vi "Tosca-MATLAB Thread.vi"   [LabVIEW 2020]
uses:
  Typedefs/Tosca-MATLAB Queue Data.ctl
types:
  T1 = typedef "Tosca-MATLAB Queue Data.ctl" = cluster{"MATLAB function":path, "Datafile":path}
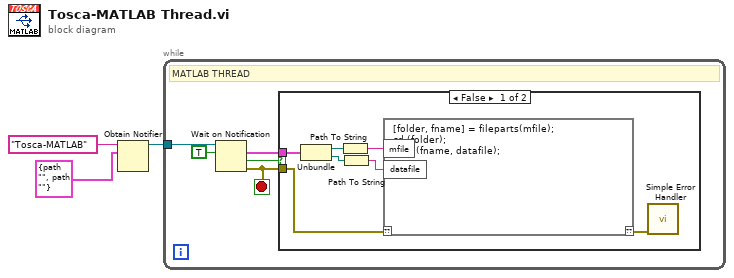
[diagram p0: block diagram]
diagram:
  n1 = Obtain Notifier(name (unnamed)="Tosca-MATLAB" ("Start"), notification data type=T1 {"MATLAB function"=path "", "Datafile"=path ""} ("Data")) -> (notifier out=w1:refnum<notifier>)  [unwired: 2 in, 2 out]
  n2 = while {
    tunnel: w1 -> [w8]
    stop <- w5 stop-if-true
    # "MATLAB THREAD"
    n3 = Wait on Notification(notifier=w8, ignore previous (F)=TRUE) -> (notification=w6:T1, timed out?=w7:bool, error out=w5:errorcluster)  [unwired: 2 in, 1 out]
    n4 = case shown="False" w7 {
      tunnel: w6 -> [w15 _]
      tunnel: w5 -> [w12 _]
      frame False {
        n5 = Unbundle(w15) -> ("MATLAB function"=w14:path, "Datafile"=w13:path)
        n6 = Path To String(path=w14) -> (string=w10:string)
        n7 = Path To String(path=w13) -> (string=w11:string)
        n8 = script code="[folder, fname] = fileparts(mfile);\ncd (folder);\nfeval(fname, datafile);"("??"=w12, "mfile"=w10, "datafile"=w11) -> ("??"=w9:errorcluster)
        n9 = call <vilib>:"Simple Error Handler.vi"("error in (no error)"=w9) -> ()  [unwired: 4 in, 5 out]
      }
      frame True {
      }
    }
  }
